vi "Calc_rhominus.vi"(10 "Q":dbl[](array[numeric]), 11 "P":dbl[](array[numeric])) -> (3 "rho+":dbl[](array[numeric]))   [LabVIEW 2018]
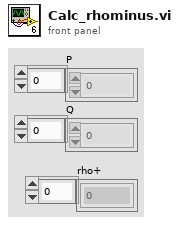
[diagram p1: front panel]
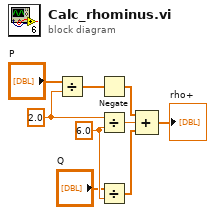
[diagram p0: block diagram]
diagram:
  w7 = 6.0
  w8 = 2.0
  n1 = Divide(x="P", y=w8) -> (x/y=w3:dbl[])
  n2 = Negate(x=w3) -> (-x=w1:dbl[])
  n3 = Divide(x=w8, y=w7) -> (x/y=w5:dbl)
  n4 = Divide(x="Q", y=w7) -> (x/y=w4:dbl[])
  n5 = Compound Arithmetic op=ADD(w1, w5, w4) -> (→"rho+":dbl[])
